vi "Step Update Map - Step Number Updated.vi"(8 "New Step Number":i32, 9 "Previous Step Number":i32, 10 "Step Update Map in":T1(c390), 11 "Settings UI in":refnum<class "Settings UI.lvclass">) -> (2 "Step Update Map out":T1(c390), 3 "Settings UI out":refnum<class "Settings UI.lvclass">)   [LabVIEW 2020, in "Output Sequencer.lvlib" / "Settings UI.lvclass"]
uses:
  Settings UI.lvclass
  Settings UI.lvclass/Settings UI.ctl
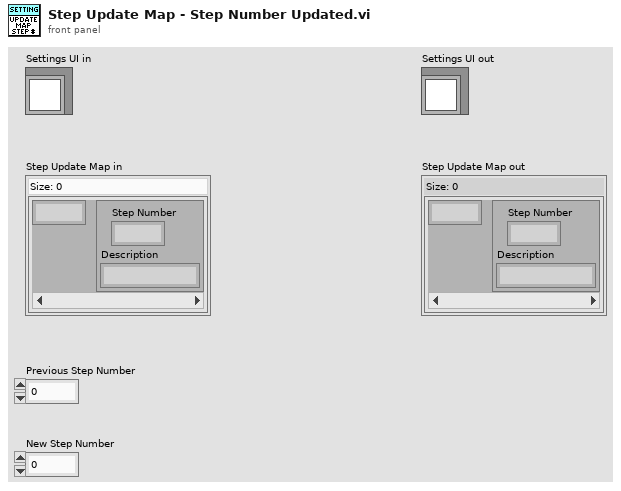
[diagram p1: front panel]
types:
  T1 = map{i32, cluster{"Step Number":i32, "Description":string}}
  T2 = typedef "Output Sequencer.lvlib/Settings UI.lvclass/Step Settings.ctl" = cluster{"Description":string, "Precondition":string, "Duration":dbl, "Mode":string, "Delay Between Values":dbl, "Analog Values":string[], "Digital Values":string[], "Postcondition":string, "On True":string, "On False":string}
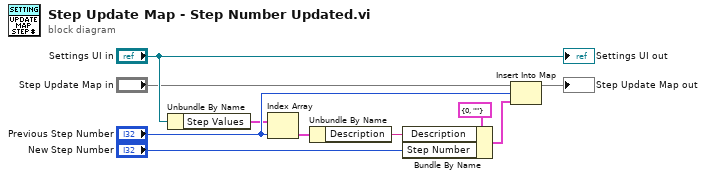
[diagram p0: block diagram]
diagram:
  n1 = Unbundle By Name("Settings UI in") -> ("Step Values"=w4:T2[])
  n2 = Index Array(array=w4, index="Previous Step Number") -> (element=w3:T2)
  n3 = Unbundle By Name(w3) -> ("Description"=w2:string)
  n4 = Bundle By Name(cluster=cluster{"Step Number":i32, "Description":string} {"Step Number"=0, "Description"=""} ("New Settings"), "Description"=w2, "Step Number"="New Step Number") -> (w5:cluster{"Step Number":i32, "Description":string})
  n5 = Insert Into Map(map in="Step Update Map in", key="Previous Step Number", value=w5) -> (map out=→"Step Update Map out":T1)  [unwired: 2 out]
  "Settings UI out" <- "Settings UI in"
